vi "CalculateDelay.vi"(8 "input valid":bool=TRUE, 9 "cos_fi":fxp<+/-,16,0>, 10 "sin fi":fxp<+/-,16,0>, 11 "Data in":fxp<+/-,16,14>[](array[numeric])=[0.0, 0.0, 0.0, 0.0]) -> (0 "output valid":bool, 3 "Data out":fxp<+/-,16,14>[](array[numeric]))   [LabVIEW 2013]
doc: "Calculates various combinations on I_in, Q_in and cos(fi) and sin(fi) to be used later to delay the output signal"
uses:
  <vilib>/rvi/FXPMathLib/FxpInterpret/XNode/nifxpmath_Interpret.xnode
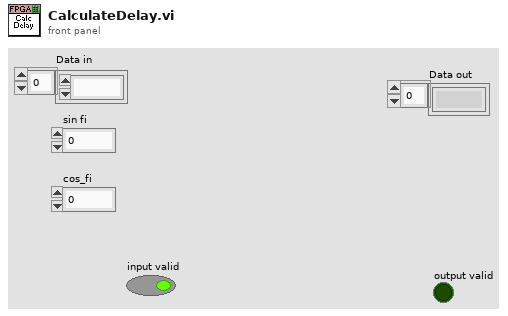
[diagram p1: front panel]
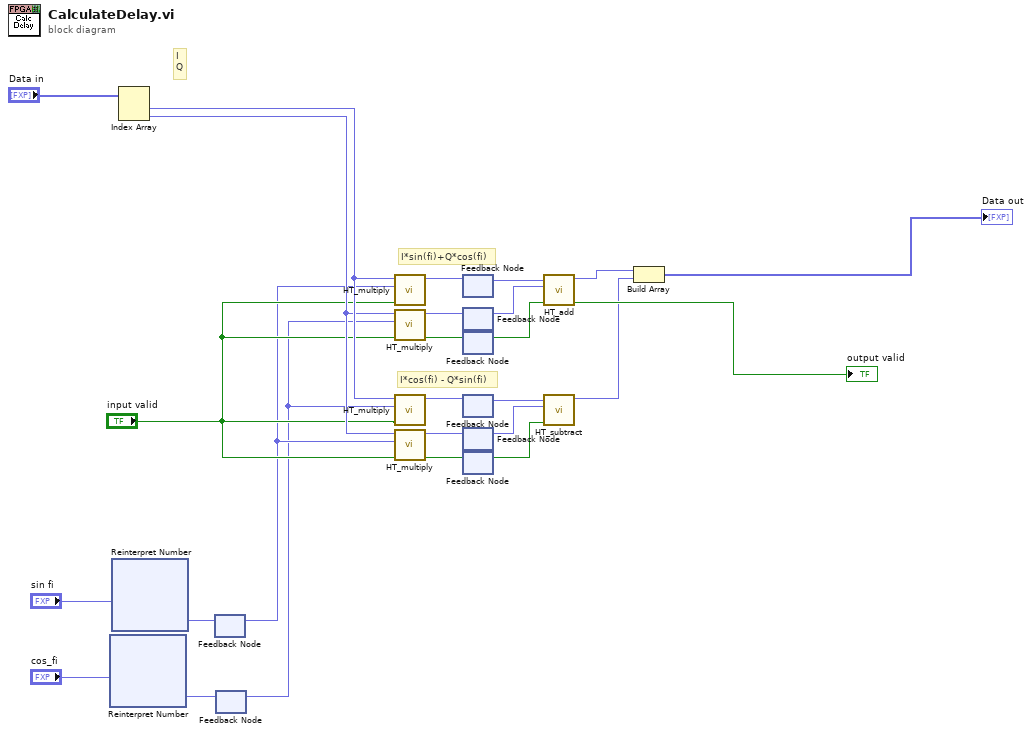
[diagram p0: block diagram]
diagram:
  # "I*cos(fi) - Q*sin(fi)"
  # "I\nQ"
  # "I*sin(fi)+Q*cos(fi)"
  n1 = xnode "Reinterpret Number"("x"="cos_fi") -> ("y"=w4:fxp<+/-,16,2>)
  n2 = xnode "Reinterpret Number"("x"="sin fi") -> ("y"=w6:fxp<+/-,16,2>)
  n3 = Index Array(array="Data in") -> (element #1=w13:fxp<+/-,16,14>, element #2=w12:fxp<+/-,16,14>)  [unwired: 2 in]
  n4 = feedback #1() -> (w5:fxp<+/-,16,2>)  [unwired: 1 in]
  n5 = feedback-in #1(w6) -> ()
  n6 = feedback #2() -> (w3:fxp<+/-,16,2>)  [unwired: 1 in]
  n7 = feedback-in #2(w4) -> ()
  n8 = call "HT_multiply.vi"("input valid"="input valid", "y"=w5, "x"=w13) -> ("x*y"=w25:fxp<+/-,16,14>)  [unwired: 7 in, 1 out]
  n9 = call "HT_multiply.vi"("input valid"="input valid", "y"=w3, "x"=w12) -> ("output valid"=w20:bool, "x*y"=w22:fxp<+/-,16,14>)  [unwired: 7 in]
  n10 = call "HT_multiply.vi"("input valid"="input valid", "y"=w3, "x"=w13) -> ("x*y"=w14:fxp<+/-,16,14>)  [unwired: 7 in, 1 out]
  n11 = call "HT_multiply.vi"("input valid"="input valid", "y"=w5, "x"=w12) -> ("output valid"=w19:bool, "x*y"=w17:fxp<+/-,16,14>)  [unwired: 7 in]
  n12 = feedback #3() -> (w24:fxp<+/-,16,14>)  [unwired: 1 in]
  n13 = feedback-in #3(w25) -> ()
  n14 = feedback #4() -> (w21:fxp<+/-,16,14>)  [unwired: 1 in]
  n15 = feedback-in #4(w22) -> ()
  n16 = feedback #5() -> (w23:bool)  [unwired: 1 in]
  n17 = feedback-in #5(w20) -> ()
  n18 = feedback #6() -> (w15:fxp<+/-,16,14>)  [unwired: 1 in]
  n19 = feedback-in #6(w14) -> ()
  n20 = feedback #7() -> (w18:fxp<+/-,16,14>)  [unwired: 1 in]
  n21 = feedback-in #7(w17) -> ()
  n22 = feedback #8() -> (w16:bool)  [unwired: 1 in]
  n23 = feedback-in #8(w19) -> ()
  n24 = call "HT_add.vi"("input valid"=w23, "y"=w21, "x"=w24) -> ("output valid"=→"output valid":bool, "x+y"=w1:fxp<+/-,16,14>)  [unwired: 7 in]
  n25 = call "HT_subtract.vi"("input valid"=w16, "y"=w18, "x"=w15) -> ("x+y"=w2:fxp<+/-,16,14>)  [unwired: 7 in, 1 out]
  n26 = Build Array(w1, w2) -> (→"Data out":fxp<+/-,16,14>[])
